vi "DIAdem Wait For Response.vi"(8 "error in (no error)":errorcluster, 9 "timeout in ms (-1)":i32=-1, 10 "Wait for Response? (f)":bool, 11 "notifier (NULL)":refnum<notifier>) -> (0 "error out":errorcluster, 1 "Timed Out?":bool, 2 "Response":string, 3 "dup notifier":refnum<notifier>)   [LabVIEW 2011]
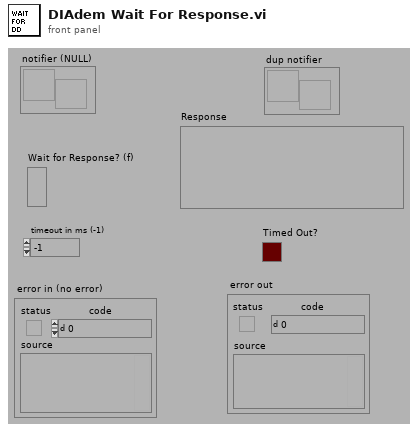
[diagram p1: front panel]
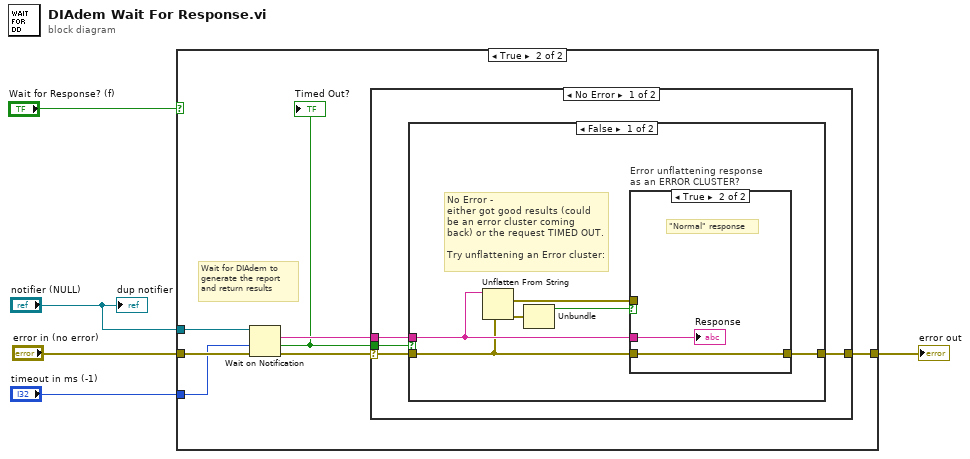
[diagram p0: block diagram]
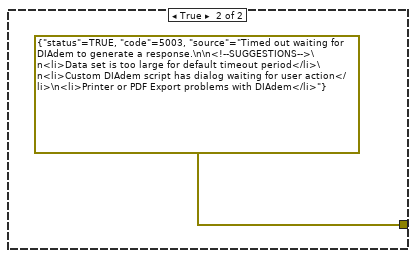
[diagram p4: hidden frame]
diagram:
  n1 = case shown="True" "Wait for Response? (f)" {
    tunnel: "notifier (NULL)" -> [_ w10]
    tunnel: "error in (no error)" -> [w6 w9]
    tunnel: [w6 w13] -> w2
    tunnel: "timeout in ms (-1)" -> [_ w8]
    frame False {
      # "Don't Wait for Completion"
    }
    frame True {
      # "Wait for DIAdem to\ngenerate the report\nand return results"
      n2 = Wait on Notification(notifier=w10, timeout in ms (-1)=w8, error in (no error)=w9) -> (notification=w12:string, timed out?=w7:bool, error out=w11:errorcluster)  [unwired: 2 out]
      "Timed Out?" <- w7
      n3 = case shown="No Error" w11 {
        selector: w11 -> [w15 w28]
        tunnel: [w17 w28] -> w13
        tunnel: w12 -> [w16 _]
        tunnel: w7 -> [w14 _]
        frame No Error {
          n4 = case shown="False" w14 {
            tunnel: [w23 errorcluster {"status"=TRUE, "code"=5003, "source"="Timed out waiting for DIAdem to generate a response.\n\n<!--SUGGESTIONS-->\n<li>Data set is too large for default timeout period</li>\n<li>Custom DIAdem script has dialog waiting for user action</li>\n<li>Printer or PDF Export problems with DIAdem</li>"} ("error in (no error)")] -> w17
            tunnel: w16 -> [w20 _]
            tunnel: w15 -> [w18 _]
            frame False {
              # "No Error -\neither got good results (could\nbe an error cluster coming\nback) or the request TIMED OUT.\n\nTry unflattening an Error cluster:"
              n5 = Unflatten From String(type=w18, binary string=w20) -> (value=w21:errorcluster, error out=w19:errorcluster)  [unwired: 1 in, 3 out]
              n6 = Unbundle(w19) -> ("status"=w22:bool)  [unwired: 2 out]
              n7 = case "Error unflattening response\nas an ERROR CLUSTER?" shown="True" w22 {
                tunnel: w18 -> [_ w26]
                tunnel: [w24 w26] -> w23
                tunnel: w20 -> [_ w25]
                tunnel: w21 -> [w24 _]
                frame False {
                  # "DD found ERROR\n\nPass into normal error\nflow."
                }
                frame True {
                  # "\"Normal\" response"
                  "Response" <- w25
                }
              }
            }
            frame True {
            }
          }
        }
        frame Error {
          # "< NOTE Timeouts DO NOT set Error Status = TRUE"
          # "There was an error.  Probably due\nto the Q being destroyed since\nuser browsed off of CGI."
        }
      }
    }
  }
  "error out" <- w2
  "dup notifier" <- "notifier (NULL)"
